vi "Update Add Run Parameters.vi"(0 "Parameters Map":map{string, string[]}(c390)) -> ()   [LabVIEW 2020, in "CIRCUS_uServices.lvlib" / "Scheduler.lvlib"]
uses:
  Scheduler.lvlib
  Add RUN Window.vi
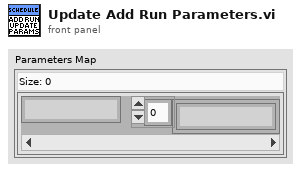
[diagram p1: front panel]
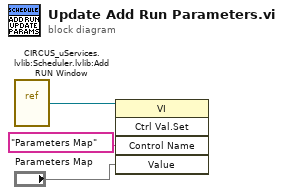
[diagram p0: block diagram]
diagram:
  n1 = vi-ref "CIRCUS_uServices.lvlib:Scheduler.lvlib:Add RUN Window.vi"() -> (w1:refnum<vi>)
  n2 = invoke class="VI" method="Ctrl Val.Set"(reference=w1, "Control Name"="Parameters Map", "Value"="Parameters Map") -> ()  [unwired: 2 in, 5 out]
